vi "MacroStagePositioning_MD.vi"() -> ()   [LabVIEW 2012]
doc: "SciScan 1.2 160622"
uses:
  CommonResource VIs/Timing/Timer Commands.ctl
  GFG/GFGnumericGet.vi
  GFG/GFG library.lvlib
panel:
  out "Error Out":errorcluster
  in  "Error In":errorcluster
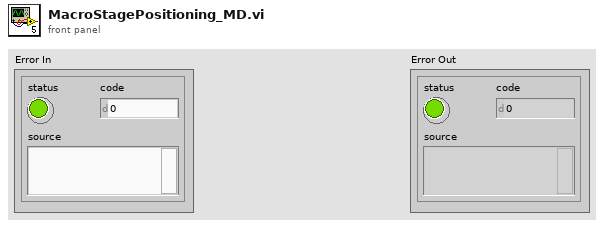
[diagram p1: front panel]
types:
  T1 = typedef "Timer Commands.ctl" = enum16{"Clear All", "Start", "Pause", "Check Time"}
  T2 = cluster{"moveXabs":dbl, "moveYabs":dbl, "moveZabs":dbl}
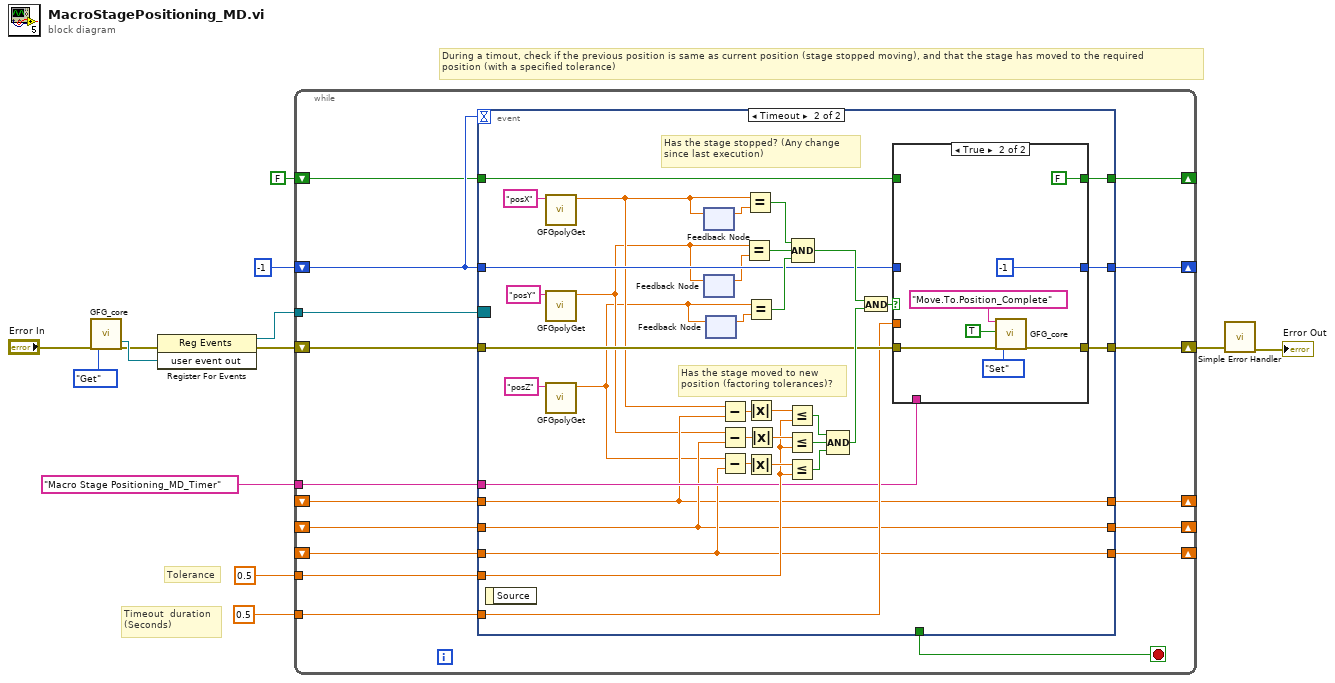
[diagram p0: block diagram]
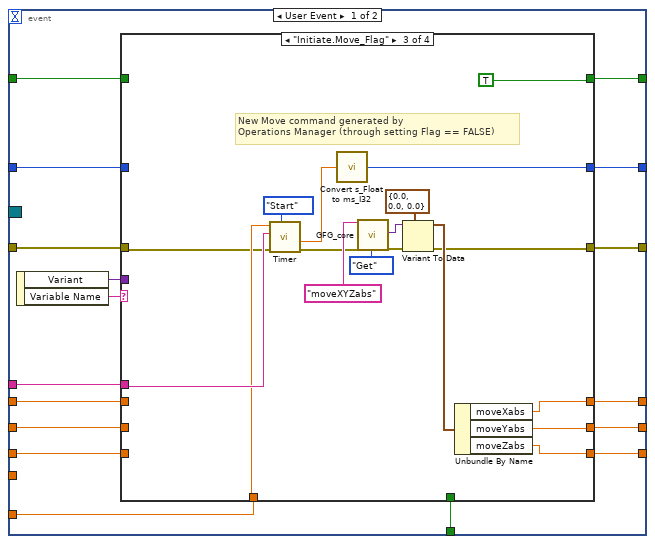
[diagram p2: hidden frame]
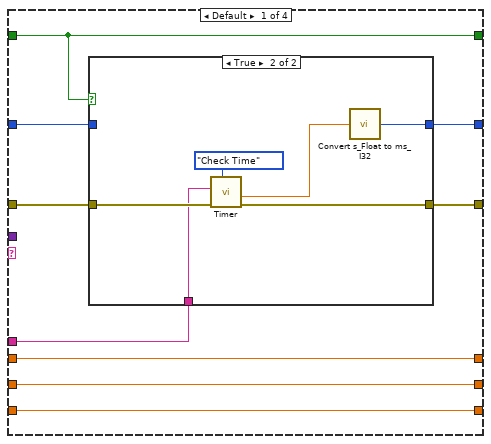
[diagram p3: hidden frame]
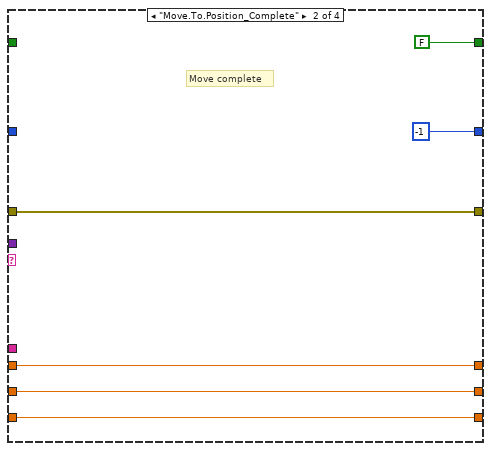
[diagram p5: hidden frame]
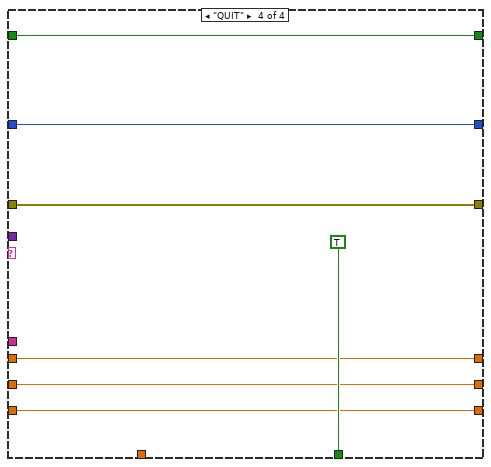
[diagram p6: hidden frame]
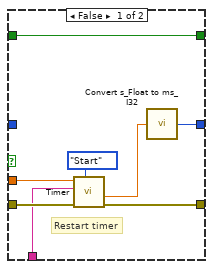
[diagram p7: hidden frame]
diagram:
  # "During a timout, check if the previous position is same as current position (stage stopped moving), and that the stage has moved to the required\nposition (with a specified tolerance)"
  # "Timeout  duration\n(Seconds)"
  # "Tolerance"
  n1 = call "GFG_core.vi"("error in (no error)"="Error In", "Action"=enum16{"Init", "Set", "Get", "Clear"}."Get") -> ("user event out"=w13:refnum<user-event>, "error out"=w9:errorcluster)  [unwired: 11 in, 5 out]
  n2 = register-events(error in=w9, w13) -> (reference out=w12:refnum<event-registration>, error out=w8:errorcluster)  [unwired: 1 in]
  n3 = while {
    tunnel: w12 -> [w30]
    shift-right: [w27] -> _
    shift-left: -1 -> [w16]
    tunnel: "Macro Stage Positioning_MD_Timer" ("VI name (Optional)") -> [w26]
    shift-right: [w25] -> w4
    shift-left: w8 -> [w28]
    tunnel: 0.5 ("Set Time IN (s)") -> [w24]
    shift-right: [w23] -> _
    shift-left: _ -> [w20]
    shift-right: [w22] -> _
    shift-left: _ -> [w19]
    shift-right: [w21] -> _
    shift-left: _ -> [w18]
    tunnel: 0.5 ("Set Time IN (s)") -> [w17]
    shift-right: [w15] -> _
    shift-left: FALSE -> [w14]
    stop <- w29 stop-if-true
    n4 = event shown="[1] Timeout" {
      selector: w30 -> [_ _]
      dyn-events: _ -> [_ _]
      timeout: w16 -> [_ _]
      tunnel: [w46 _] -> w29
      tunnel: w28 -> [w44 w110]
      tunnel: [w43 w111] -> w27
      tunnel: w16 -> [w42 w112]
      tunnel: w26 -> [w33 w107]
      tunnel: [w41 w109] -> w25
      tunnel: w24 -> [w40 w108]
      tunnel: [w39 w106] -> w23
      tunnel: [w37 w105] -> w22
      tunnel: [w35 w104] -> w21
      tunnel: w20 -> [w38 w106]
      tunnel: w19 -> [w36 w105]
      tunnel: w18 -> [w34 w104]
      tunnel: w17 -> [_ w122]
      tunnel: [w32 w96] -> w15
      tunnel: w14 -> [w31 w97]
      event User Event {
        n5 = event-data() -> ("Variant"=w45:variant, "Variable Name"=w47:string)  [unwired: 1 in]
        n6 = case shown="\"Initiate.Move_Flag\"" w47 {
          tunnel: [_ _ _ TRUE] -> w46
          tunnel: w45 -> [_ _ _ _]
          tunnel: w44 -> [w55 w65 w72 w93]
          tunnel: [w56 -1 ("milliseconds OUT (I32)") w71 w94] -> w43
          tunnel: w42 -> [w48 _ _ w94]
          tunnel: [w54 w65 w78 w93] -> w41
          tunnel: w40 -> [_ _ w73 _]
          tunnel: [w51 w69 w75 w92] -> w39
          tunnel: w38 -> [w51 w69 _ w92]
          tunnel: [w52 w68 w76 w91] -> w37
          tunnel: w36 -> [w52 w68 _ w91]
          tunnel: [w53 w67 w77 w90] -> w35
          tunnel: w34 -> [w53 w67 _ w90]
          tunnel: w33 -> [w50 _ w74 _]
          tunnel: [w49 FALSE TRUE w89] -> w32
          tunnel: w31 -> [w49 _ _ w89]
          frame Default {
            n7 = case shown="True" w49 {
              tunnel: [w58 w62] -> w56
              tunnel: w55 -> [w57 w61]
              tunnel: [w57 w60] -> w54
              tunnel: w50 -> [_ w59]
              tunnel: w48 -> [w58 _]
              frame False {
                # "Don't update timeout if Move not in progress\n(i.e. Timeout value == -1)"
              }
              frame True {
                n8 = call "Timer.vi"("Timer Command"=Timer_Commands."Check Time", "Error In"=w61, "VI name (Optional)"=w59) -> ("Error Out"=w60:errorcluster, "Remaining Time (s)"=w63:dbl)  [unwired: 3 in, 4 out]
                n9 = call "Convert s_Float to ms_I32.vi"("Seconds IN (Float)"=w63) -> ("milliseconds OUT (I32)"=w62:i32)
              }
            }
          }
          frame "Move.To.Position_Complete" {
            # "Move complete"
          }
          frame "Initiate.Move_Flag" {
            # "New Move command generated by \nOperations Manager (through setting Flag == FALSE)"
            n10 = call "Timer.vi"("Timer Command"=Timer_Commands."Start", "Error In"=w72, "VI name (Optional)"=w74, "Set Time IN (s)"=w73) -> ("Error Out"=w84:errorcluster, "Remaining Time (s)"=w87:dbl)  [unwired: 2 in, 4 out]
            n11 = call "Convert s_Float to ms_I32.vi"("Seconds IN (Float)"=w87) -> ("milliseconds OUT (I32)"=w71:i32)
            n12 = call "GFG_core.vi"("Variable Name in"="moveXYZabs", "error in (no error)"=w84, "Action"=enum16{"Init", "Set", "Get"}."Get") -> ("Variant Out"=w82:variant, "error out"=w81:errorcluster)  [unwired: 10 in, 5 out]
            n13 = Variant To Data(error in=w81, type=T2 {"moveXabs"=0.0, "moveYabs"=0.0, "moveZabs"=0.0} ("output cluster"), Variant=w82) -> (data=w80:T2, error out=w78:errorcluster)
            n14 = Unbundle By Name(w80) -> ("moveXabs"=w77:dbl, "moveYabs"=w76:dbl, "moveZabs"=w75:dbl)
          }
          frame "QUIT" {
          }
        }
      }
      event Timeout {
        # "Has the stage moved to new\nposition (factoring tolerances)?"
        # "Has the stage stopped? (Any change since last execution)"
        n15 = event-data() -> ()  [unwired: 1 in, 1 out]
        n16 = call-poly "GFGpolyGet.vi"("Variable Name in"="posX") -> ("Numeric"=w103:dbl)  [unwired: 8 in, 2 out]
        n17 = call-poly "GFGpolyGet.vi"("Variable Name in"="posY") -> ("Numeric"=w101:dbl)  [unwired: 8 in, 2 out]
        n18 = call-poly "GFGpolyGet.vi"("Variable Name in"="posZ") -> ("Numeric"=w99:dbl)  [unwired: 8 in, 2 out]
        n19 = feedback-in #1(w103) -> ()
        n20 = feedback #1() -> (w102:dbl)  [unwired: 1 in]
        n21 = feedback #2() -> (w100:dbl)  [unwired: 1 in]
        n22 = feedback-in #2(w101) -> ()
        n23 = feedback #3() -> (w98:dbl)  [unwired: 1 in]
        n24 = feedback-in #3(w99) -> ()
        n25 = Subtract(x=w103, y=w104) -> (x-y=w128:dbl)
        n26 = Subtract(x=w101, y=w105) -> (x-y=w126:dbl)
        n27 = Subtract(x=w99, y=w106) -> (x-y=w127:dbl)
        n28 = Equal?(x=w101, y=w100) -> (x = y?=w118:bool)
        n29 = Equal?(x=w103, y=w102) -> (x = y?=w117:bool)
        n30 = Equal?(x=w99, y=w98) -> (x = y?=w116:bool)
        n31 = Absolute Value(x=w128) -> (abs(x)=w123:dbl)
        n32 = Absolute Value(x=w127) -> (abs(x)=w125:dbl)
        n33 = Absolute Value(x=w126) -> (abs(x)=w124:dbl)
        n34 = Less Or Equal?(x=w123, y=w122) -> (x <= y?=w120:bool)
        n35 = Less Or Equal?(x=w124, y=w122) -> (x <= y?=w121:bool)
        n36 = Less Or Equal?(x=w125, y=w122) -> (x <= y?=w119:bool)
        n37 = Compound Arithmetic op=AND(w117, w118, w116) -> (w114:bool)
        n38 = Compound Arithmetic op=AND(w120, w121, w119) -> (w115:bool)
        n39 = And(x=w114, y=w115) -> (x .and. y?=w113:bool)
        n40 = case shown="True" w113 {
          tunnel: w112 -> [_ _]
          tunnel: [w136 -1 ("milliseconds OUT (I32)")] -> w111
          tunnel: w110 -> [w137 w142]
          tunnel: [w135 w141] -> w109
          tunnel: w108 -> [w134 _]
          tunnel: w107 -> [w133 _]
          tunnel: w97 -> [w132 _]
          tunnel: [w132 FALSE] -> w96
          frame False {
            # "Restart timer"
            n41 = call "Timer.vi"("Timer Command"=Timer_Commands."Start", "Error In"=w137, "VI name (Optional)"=w133, "Set Time IN (s)"=w134) -> ("Error Out"=w135:errorcluster, "Remaining Time (s)"=w138:dbl)  [unwired: 2 in, 4 out]
            n42 = call "Convert s_Float to ms_I32.vi"("Seconds IN (Float)"=w138) -> ("milliseconds OUT (I32)"=w136:i32)
          }
          frame True {
            n43 = call "GFG_core.vi"("Variable Name in"="Move.To.Position_Complete" ("VI name (Optional)"), "Variant in"=TRUE, "error in (no error)"=w142, "Action"=enum16{"Init", "Set", "Get", "Clear"}."Set") -> ("error out"=w141:errorcluster)  [unwired: 9 in, 6 out]
          }
        }
      }
    }
  }
  n44 = call <vilib>:"Simple Error Handler.vi"("error in (no error)"=w4) -> ("error out"=→"Error Out":errorcluster)  [unwired: 4 in, 4 out]
